vi "Read Power FIFO Direct Dispatch.vi"(8 "error in (no error)":errorcluster, 9 "Timeout (ms)":i32, 10 "Data in":T1[](array[typedef])=[{"measurement"=[], "dT"=0.0, "Timestamp"=0, "Read Lock"=FALSE}, {"measurement"=[], "dT"=0.0, "Timestamp"=0, "Read Lock"=FALSE}], 11 "CIFTag in":refnum<class "CIFChannels.lvclass">) -> (0 "error out":errorcluster, 1 "timed out?":bool, 2 "Data out":T1[](array[typedef]), 3 "CIFTag out":refnum<class "CIF_NIChn_Fifo_Power.lvclass">, 4 "Header":T2)   [LabVIEW 2021, in "CIF_NIChn_Fifo_Power.lvclass"]
uses:
  CIF_NIChn_Fifo_Power.lvclass
  D:/dev/Packages/Channel_Manager/src/CIFChannels/CIFChannels.lvclass
  D:/dev/Packages/Channel_Manager/src/CIF_NIChn/NIChn/CIF_NIChn.lvclass
  ChannelCommon/typedef/FIFO Header.ctl
  CIFChannels/CIFChannels.lvclass
  ChannelCommon/typedef/Datatype Waveform.ctl
  CIFChannels/CIFChannels.lvclass/CIFChannels.ctl
  CIFChannels/Typedef/Channel State.ctl
  CIFChannels/Typedef/Direction.ctl
  NIChn/CIF_NIChn.lvclass/CIF_NIChn.ctl
  CIFChannels/Accessors/Read Channel State.vi
  CIFChannels/Accessors/Read Direction.vi
  ChannelCommon/Utilities/Unflatten Header.vi
  <vilib>/CIF Foundation/CIF Utilities/DataTypes/Unflatten I64.vi
  <vilib>/CIF Foundation/CIF Utilities/DataTypes/Unflatten U64.vi
  <vilib>/CIF Foundation/CIF Channels/CIFChannels/Top Level/Advanced/Read U8 FIFO as Dbl Array.vi
  ChannelCommon/Utilities/Add Error.vi
  <vilib>/CIF Foundation/CIF Channels/CIFChannels/Top Level/Read U8 Array.vi/4bc1c15b-36ab-481f-b8dd-c64075ce723a.vi
  <vilib>/CIF Foundation/CIF Channels/CIFChannels/Top Level/Read U8 Array.vi/d83cb72b-7713-41fc-a3d1-682de79cf574.vi
  <vilib>/CIF Foundation/CIF Channels/CIFChannels/SubVIs/Get dll Path.vi
  <vilib>/CIF Foundation/CIF Channels/CIFChannels/SubVIs/Get Requested Size.vi
  <vilib>/CIF Foundation/CIF Channels/CIFChannels/Top Level/Advanced/Read U8 FIFO as Dbl Array.vi/4bc1c15b-36ab-481f-b8dd-c64075ce723a.vi
  <vilib>/CIF Foundation/CIF Channels/CIFChannels/Top Level/Advanced/Read U8 FIFO as Dbl Array.vi/d83cb72b-7713-41fc-a3d1-682de79cf574.vi
  <vilib>/CIF Foundation/CIF Utilities/Errors/Append Error Location.vi
  NIChn/CIF_NIChn.lvclass
  <vilib>/CIF Foundation/CIF Channels/CIFChannels/CIFChannelCore.lvlib
  ChannelCommon/ChannelCommon.lvlib
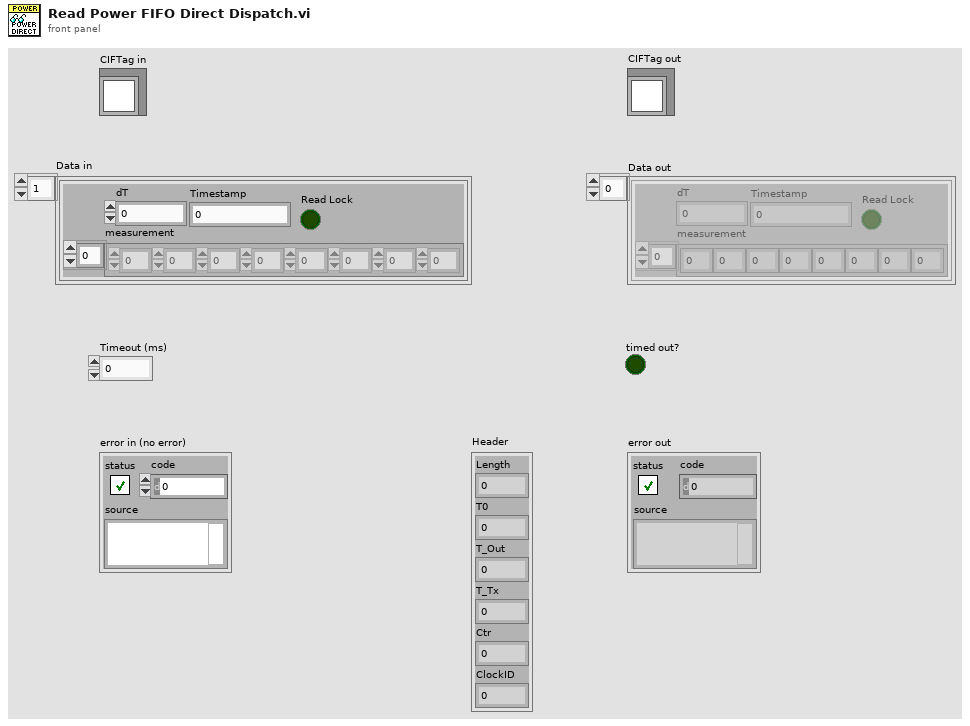
[diagram p1: front panel]
types:
  T1 = typedef "ChannelCommon.lvlib/Datatype Waveform.ctl" = cluster{"measurement":dbl[], "dT":dbl, "Timestamp":i64, "Read Lock":bool}
  T2 = typedef "ChannelCommon.lvlib/FIFO Header.ctl" = cluster{"Length":u64, "T0":i64, "T_Out":i64, "T_Tx":i64, "Ctr":u64, "ClockID":u8}
  T3 = typedef "CIFChannels.lvclass/Channel State.ctl" = enum16{"Creating", "Disconnected", "Connecting", "Connected", "Destroyed"}
  T4 = typedef "CIFChannels.lvclass/Direction.ctl" = enum16{"Publisher", "Subscriber"}
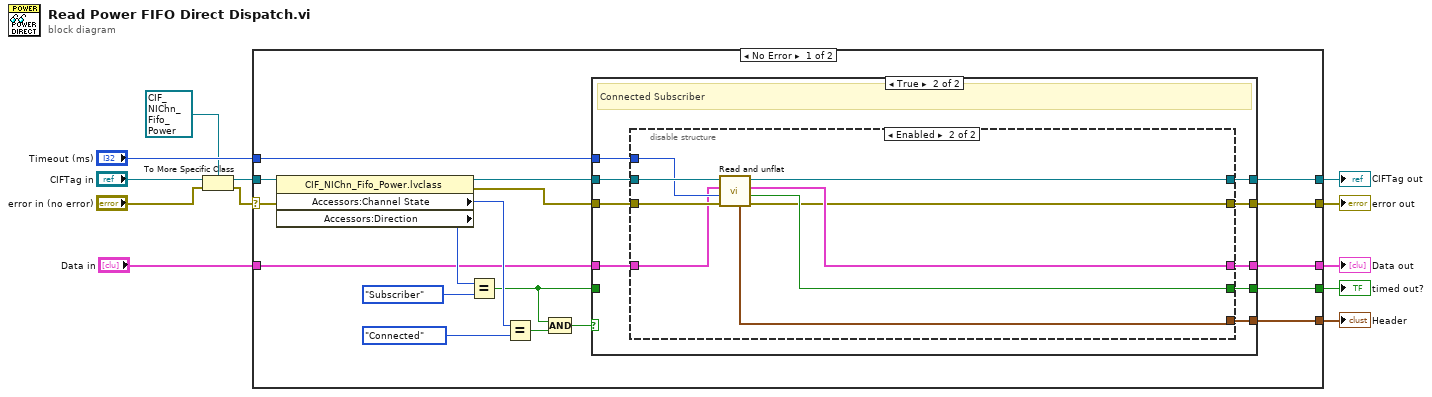
[diagram p0: block diagram]
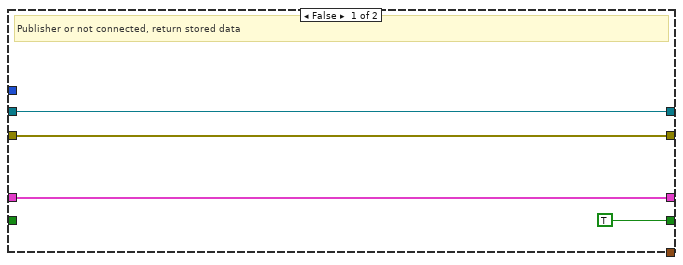
[diagram p2: hidden frame]
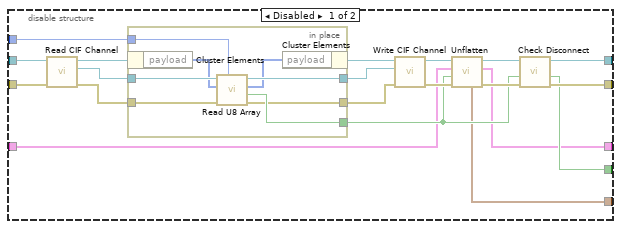
[diagram p3: hidden frame]
diagram:
  n1 = To More Specific Class(target class=refnum<class "CIF_NIChn_Fifo_Power.lvclass"> refnum ("CIFTag in"), reference="CIFTag in", error in="error in (no error)") -> (specific class reference=w5:refnum<class "CIF_NIChn_Fifo_Power.lvclass">, error out=w4:errorcluster)
  n2 = case shown="No Error" w4 {
    selector: w4 -> [w27 w83]
    tunnel: [w16 w83] -> w12
    tunnel: [w17 w82] -> w11
    tunnel: w5 -> [w28 w82]
    tunnel: [w30 _] -> w10
    tunnel: [w29 w81] -> w2
    tunnel: "Timeout (ms)" -> [w15 _]
    tunnel: [w14 _] -> w8
    tunnel: "Data in" -> [w13 w81]
    frame No Error {
      n3 = property class="CIF_NIChn_Fifo_Power.lvclass"(reference=w28, error in=w27) -> (reference out=w26:refnum<class "CIF_NIChn_Fifo_Power.lvclass">, error out=w25:errorcluster, "Accessors:Channel State"=w22:T3, "Accessors:Direction"=w24:T4)
      n4 = Equal?(x=w24, y=Direction."Subscriber") -> (x = y?=w18:bool)
      n5 = Equal?(x=w22, y=Channel_State."Connected") -> (x = y?=w20:bool)
      n6 = Compound Arithmetic op=AND(w18, w20) -> (w19:bool)
      n7 = case shown="True" w19 {
        tunnel: [TRUE ("timeout out") w39] -> w30
        tunnel: [w31 w37] -> w29
        tunnel: w25 -> [w33 w42]
        tunnel: w26 -> [w34 w43]
        tunnel: w18 -> [_ _]
        tunnel: [w34 w41] -> w17
        tunnel: [w33 w40] -> w16
        tunnel: w15 -> [_ w38]
        tunnel: [_ w36] -> w14
        tunnel: w13 -> [w31 w35]
        frame False {
          # "Publisher or not connected, return stored data"
        }
        frame True {
          # "Connected Subscriber"
          n8 = disable-structure shown="Enabled" {
            disable-tunnel: w43 -> [w63 w80]
            disable-tunnel: w42 -> [w62 w79]
            disable-tunnel: [w61 w72] -> w41
            disable-tunnel: [w60 w73] -> w40
            disable-tunnel: [w53 w75] -> w39
            disable-tunnel: w38 -> [w52 w78]
            disable-tunnel: [w46 w74] -> w37
            disable-tunnel: [w45 w76] -> w36
            disable-tunnel: w35 -> [w44 w77]
            frame Disabled {
              n9 = call "Read CIF Channel.vi"("error in (no error)"=w62, "CIFTag in"=w63) -> ("error out"=w57:errorcluster, "CIF Channel"=w58:refnum<k21>, "CIFTag out"=w59:refnum<class "CIF_NIChn_Fifo_Power.lvclass">)  [unwired: 7 in]
              n10 = in-place {
                in-place-border: [w69] -> w47
                in-place-border: w58 -> [w71]
                in-place-border: w57 -> [w70]
                in-place-border: [w68] -> w54
                in-place-border: [w67] -> w55
                in-place-border: w52 -> [w66]
                n11 = in-place-cluster #1(w59) -> ("payload"=w65:u8[])
                n12 = call <vilib>:"Read U8 Array.vi"("Timeout (ms)"=w66, "error in"=w70, "U8 Array in"=w65, "CIF Channel in"=w71) -> ("error out"=w67:errorcluster, "Timed out?"=w69:bool, "U8 Array out"=w64:u8[], "CIF Channel out"=w68:refnum<k21>)  [unwired: 4 in]
                n13 = in-place-cluster #1("payload"=w64) -> (w56:refnum<class "CIF_NIChn_Fifo_Power.lvclass">)
              }
              n14 = call "Write CIF Channel.vi"("error in (no error)"=w55, "CIF Channel"=w54, "CIFTag in"=w56) -> ("error out"=w50:errorcluster, "CIFTag out"=w51:refnum<class "CIF_NIChn_Fifo_Power.lvclass">)  [unwired: 7 in]
              n15 = call "Unflatten.vi"("error in (no error)"=w50, "timeout in"=w47, "Data in"=w44, "CIFFifoCAN in"=w51) -> ("error out"=w48:errorcluster, "Data out"=w46:T1[], "CIFFifoCAN out"=w49:refnum<class "CIF_NIChn_Fifo_Power.lvclass">, "Header"=w45:T2)  [unwired: 4 in]
              n16 = call "Check Disconnect.vi"("error in (no error)"=w48, "timeout in"=w47, "CIFTag in"=w49) -> ("error out"=w60:errorcluster, "timeout out"=w53:bool, "CIFTag out"=w61:refnum<class "CIF_NIChn_Fifo_Power.lvclass">)  [unwired: 5 in, 1 out]
            }
            frame Enabled {
              n17 = call "Read and unflat.vi"("error in (no error)"=w79, "Timeout (ms)"=w78, "Data in in"=w77, "CIF_NIChn_Fifo_Power in"=w80) -> ("error out"=w73:errorcluster, "Timed out?"=w75:bool, "Data out"=w74:T1[], "CIF_NIChn_Fifo_Power out"=w72:refnum<class "CIF_NIChn_Fifo_Power.lvclass">, "Header out"=w76:T2)  [unwired: 3 in]
            }
          }
        }
      }
    }
    frame Error {
    }
  }
  "error out" <- w12
  "CIFTag out" <- w11
  "timed out?" <- w10
  "Header" <- w8
  "Data out" <- w2
